vi "8通道控制_lock_in.vi"() -> ()   [LabVIEW 2021]
uses:
  <vilib>/Utility/error.llb/DialogType.ctl
  <vilib>/DAQmx/write.llb/DAQmx Write (Digital 2D U8 NChan NSamp).vi
  <vilib>/DAQmx/write.llb/DAQmx Write (Digital 2D U32 NChan NSamp).vi
  <vilib>/DAQmx/create/channels.llb/DAQmx Create Channel (DO-Digital Output).vi
  <vilib>/DAQmx/configure/timing.llb/DAQmx Timing (Sample Clock).vi
  <vilib>/DAQmx/miscellaneous.llb/DAQmx Fill In Error Info.vi
  <vilib>/DAQmx/configure/trigger.llb/DAQmx Start Trigger (Digital Edge).vi
  <vilib>/Utility/file.llb/Write Delimited Spreadsheet (DBL).vi
panel:
  out "error out":errorcluster
  out "写入时间（s)":dbl
  in  "采样率":dbl=10000000.0
  in  "保存总控件":bool
  in  "读取总控件":bool
  in  "Tab Control 2":enum32{"数字信号控制", "模拟信号控制"}(tab)
  out "运行状态-LED":bool
  out "运行状态":string
  in  "开始运行":bool
  in  "停止循环":bool
  in  "总时间 (ms)":dbl=100.0
  out "单通道总采样点":dbl=100000.0
  in  "结束运行":bool
  out "已运行时间 (s)":dbl
  in  "读取数字控件":bool
  in  "保存数字控件":bool
  in  "Port 0_0":T1
  out "运行状态1":bool
  in  "读取模拟控件":bool
  in  "保存模拟控件":bool
  in  "start":bool
  in  "stop":bool
  in  "Input":T2={"Digital Start Trigger Source 4"="/Dev1/PFI0", "Digital Start Trigger Edge 4"=10280, "min volt (V)"=-5.0, "max volt (V)"=5.0, "rate"=100000.0, "device name"="Dev1", "Formula In"=[], "Total time (s)"=0.0} {"rate" format="%0.2f"; "max volt (V)" format="%0.2f"; "min volt (V)" format="%0.2f"; "Digital Start Trigger Edge 4" items=["Rising"=10280, "Falling"=10171]}
  out "Output":T3={"Actual Rate"=0.0, "Actual SampPerChan"=0.0, "Mixed Signal Graph"=[], "模拟隔离器连接状态"="未连接模拟隔离器"}
  # "BEC时序控制程序"
  # "中山大学 量子工程与精密测量实验室 CPT信号控制系统"
  # "操作说明：\n1. 设置总时间和合适的采样率；\n2. 输入正数代表高电平的持续时间，负数对应低电平的持续时间。如少于总时间，之后默认为低电平；\n3. 可根据需要，拖动输入栏增加输入的时序数量；\n4. 模拟信号采用硬件触发，需将其中一个TTL信号（默认为P0.0）接入板卡的PFI0。\n5. 保存数据"
  # "AO Trigger"
  # "CPT/Probe"
  # "780"
  # "795"
  # "MOT-B"
  # "CCD"
  # "Bias-B"
  # "AI Trigger"
  # "1、Formula In 中 sample 为各个函数的持续时间\n2、Total time 为总时间，必须大于 sample 之和\n3、min volt 和 max volt 默认±10V\n4、rate 为采样率，即时钟频率\n5、device name 为选择的板卡，可选为 Dev1\n6、Source 为接受触发的端口，Edge 为触发类型"
  # "In0：780 VCO 幅值（初始 0.6）\nIn1：780 VCO 频率（初始 0.7）"
  # "Actual Rate 显示实际的时钟\n频率。Actual SampPer Chan显示\n每次采样的总样本点数。"
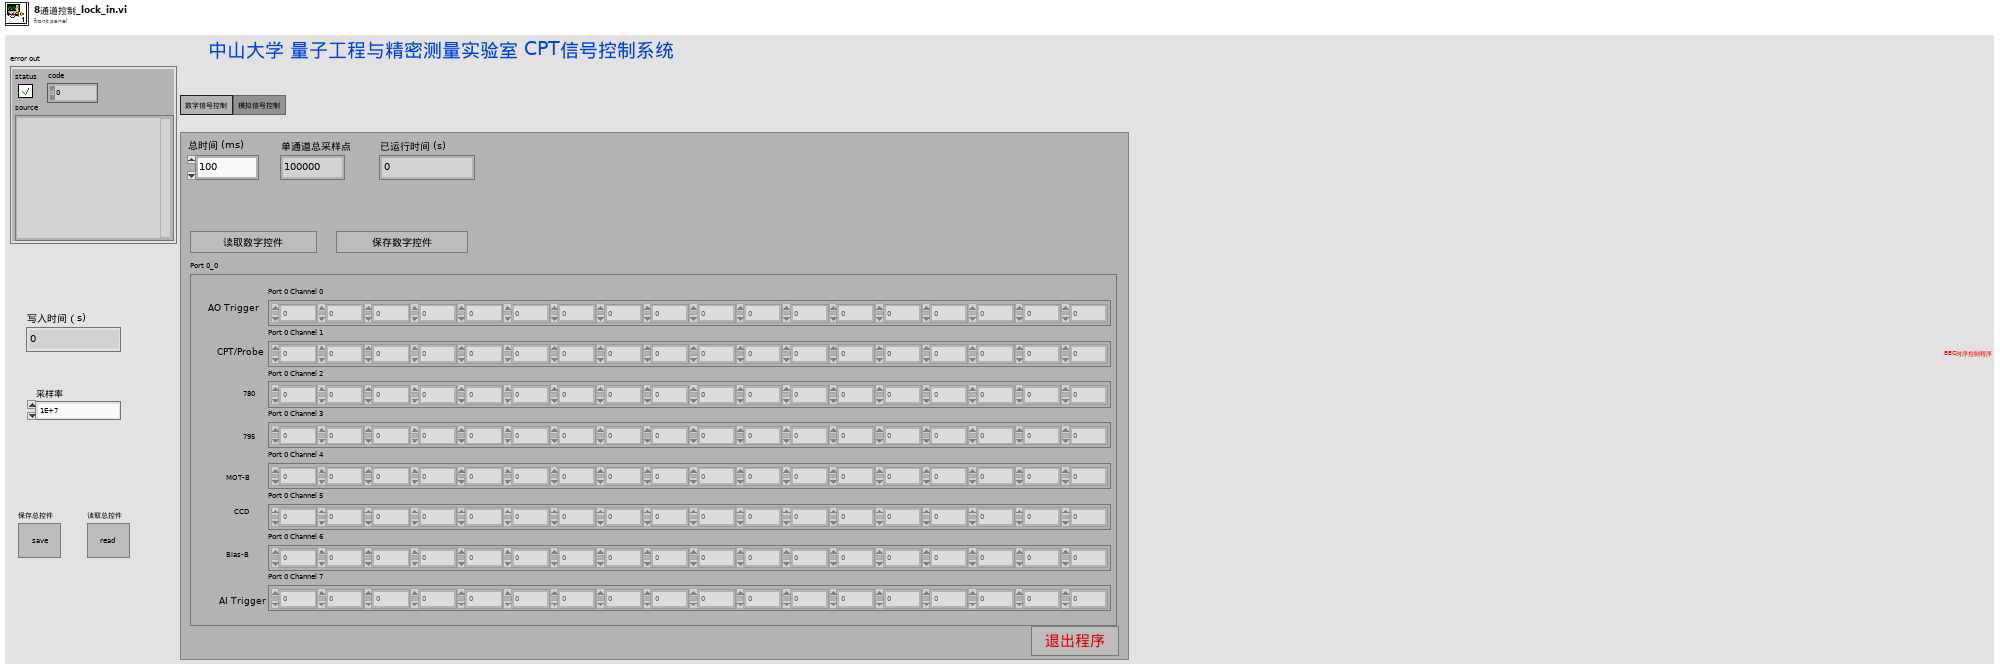
[diagram p1: front panel]
types:
  T1 = cluster{"Port 0 Channel 1":dbl[], "Port 0 Channel 2":dbl[], "Port 0 Channel 3":dbl[], "Port 0 Channel 4":dbl[], "Port 0 Channel 5":dbl[], "Port 0 Channel 6":dbl[], "Port 0 Channel 7":dbl[], "Port 0 Channel 0":dbl[]}
  T2 = cluster{"Digital Start Trigger Source 4":tag, "Digital Start Trigger Edge 4":i32, "min volt (V)":dbl, "max volt (V)":dbl, "rate":dbl, "device name":tag, "Formula In":cluster{" Sample1(s)":dbl, "formula1":string, "Sample2":dbl, "formula2":string, "Sample3":dbl, "formula3":string, "Sample4":dbl, "formula4":string}[], "Total time (s)":dbl}
  T3 = cluster{"Actual Rate":dbl, "Actual SampPerChan":dbl, "Mixed Signal Graph":waveform(dbl)[], "模拟隔离器连接状态":string}
  T4 = enum8{"Enabled", "Disabled", "Disabled and Grayed Out"}
  T5 = typedef "DialogType.ctl" = u16
  T6 = cluster{dbl[], dbl[], dbl[], dbl[], dbl[], dbl[], dbl[], dbl[]}
  T7 = cluster{"Digital Start Trigger Source 4":tag, "Digital Start Trigger Edge 4":i32, "minimum value":dbl, "maximum value":dbl, "rate":dbl, "device name":tag, "formular in":cluster{"Sample1":dbl, "formula1":string, "Sample2":dbl, "formula2":string, "Sample3":dbl, "formula3":string, "Sample4":dbl, "formula4":string}[], "Total time":dbl}
  T8 = cluster{"总时间 (ms)":dbl, "Port 0_0":cluster{"Port 0 Channel 1":dbl[], "Port 0 Channel 2":dbl[], "Port 0 Channel 3":dbl[], "Port 0 Channel 4":dbl[], "Port 0 Channel 5":dbl[], "Port 0 Channel 6":dbl[], "Port 0 Channel 7":dbl[], "Port 0 Channel 0":dbl[]}, "output":cluster{"Digital Start Trigger Source 4":string, "Digital Start Trigger Edge 4":string, "minimum value":dbl, "maximum value":dbl, "rate":dbl, "device name":string, "Total time":dbl, "Formula In":cluster{" Sample1(s)":dbl, "formula1":string, "Sample2":dbl, "formula2":string, "Sample3":dbl, "formula3":string, "Sample4":dbl, "formula4":string}[]}}
  T9 = cluster{"Digital Start Trigger Source 4":string, "Digital Start Trigger Edge 4":string, "minimum value":dbl, "maximum value":dbl, "rate":dbl, "device name":string, "Total time":dbl, "Formula In":cluster{" Sample1(s)":dbl, "formula1":string, "Sample2":dbl, "formula2":string, "Sample3":dbl, "formula3":string, "Sample4":dbl, "formula4":string}[]}
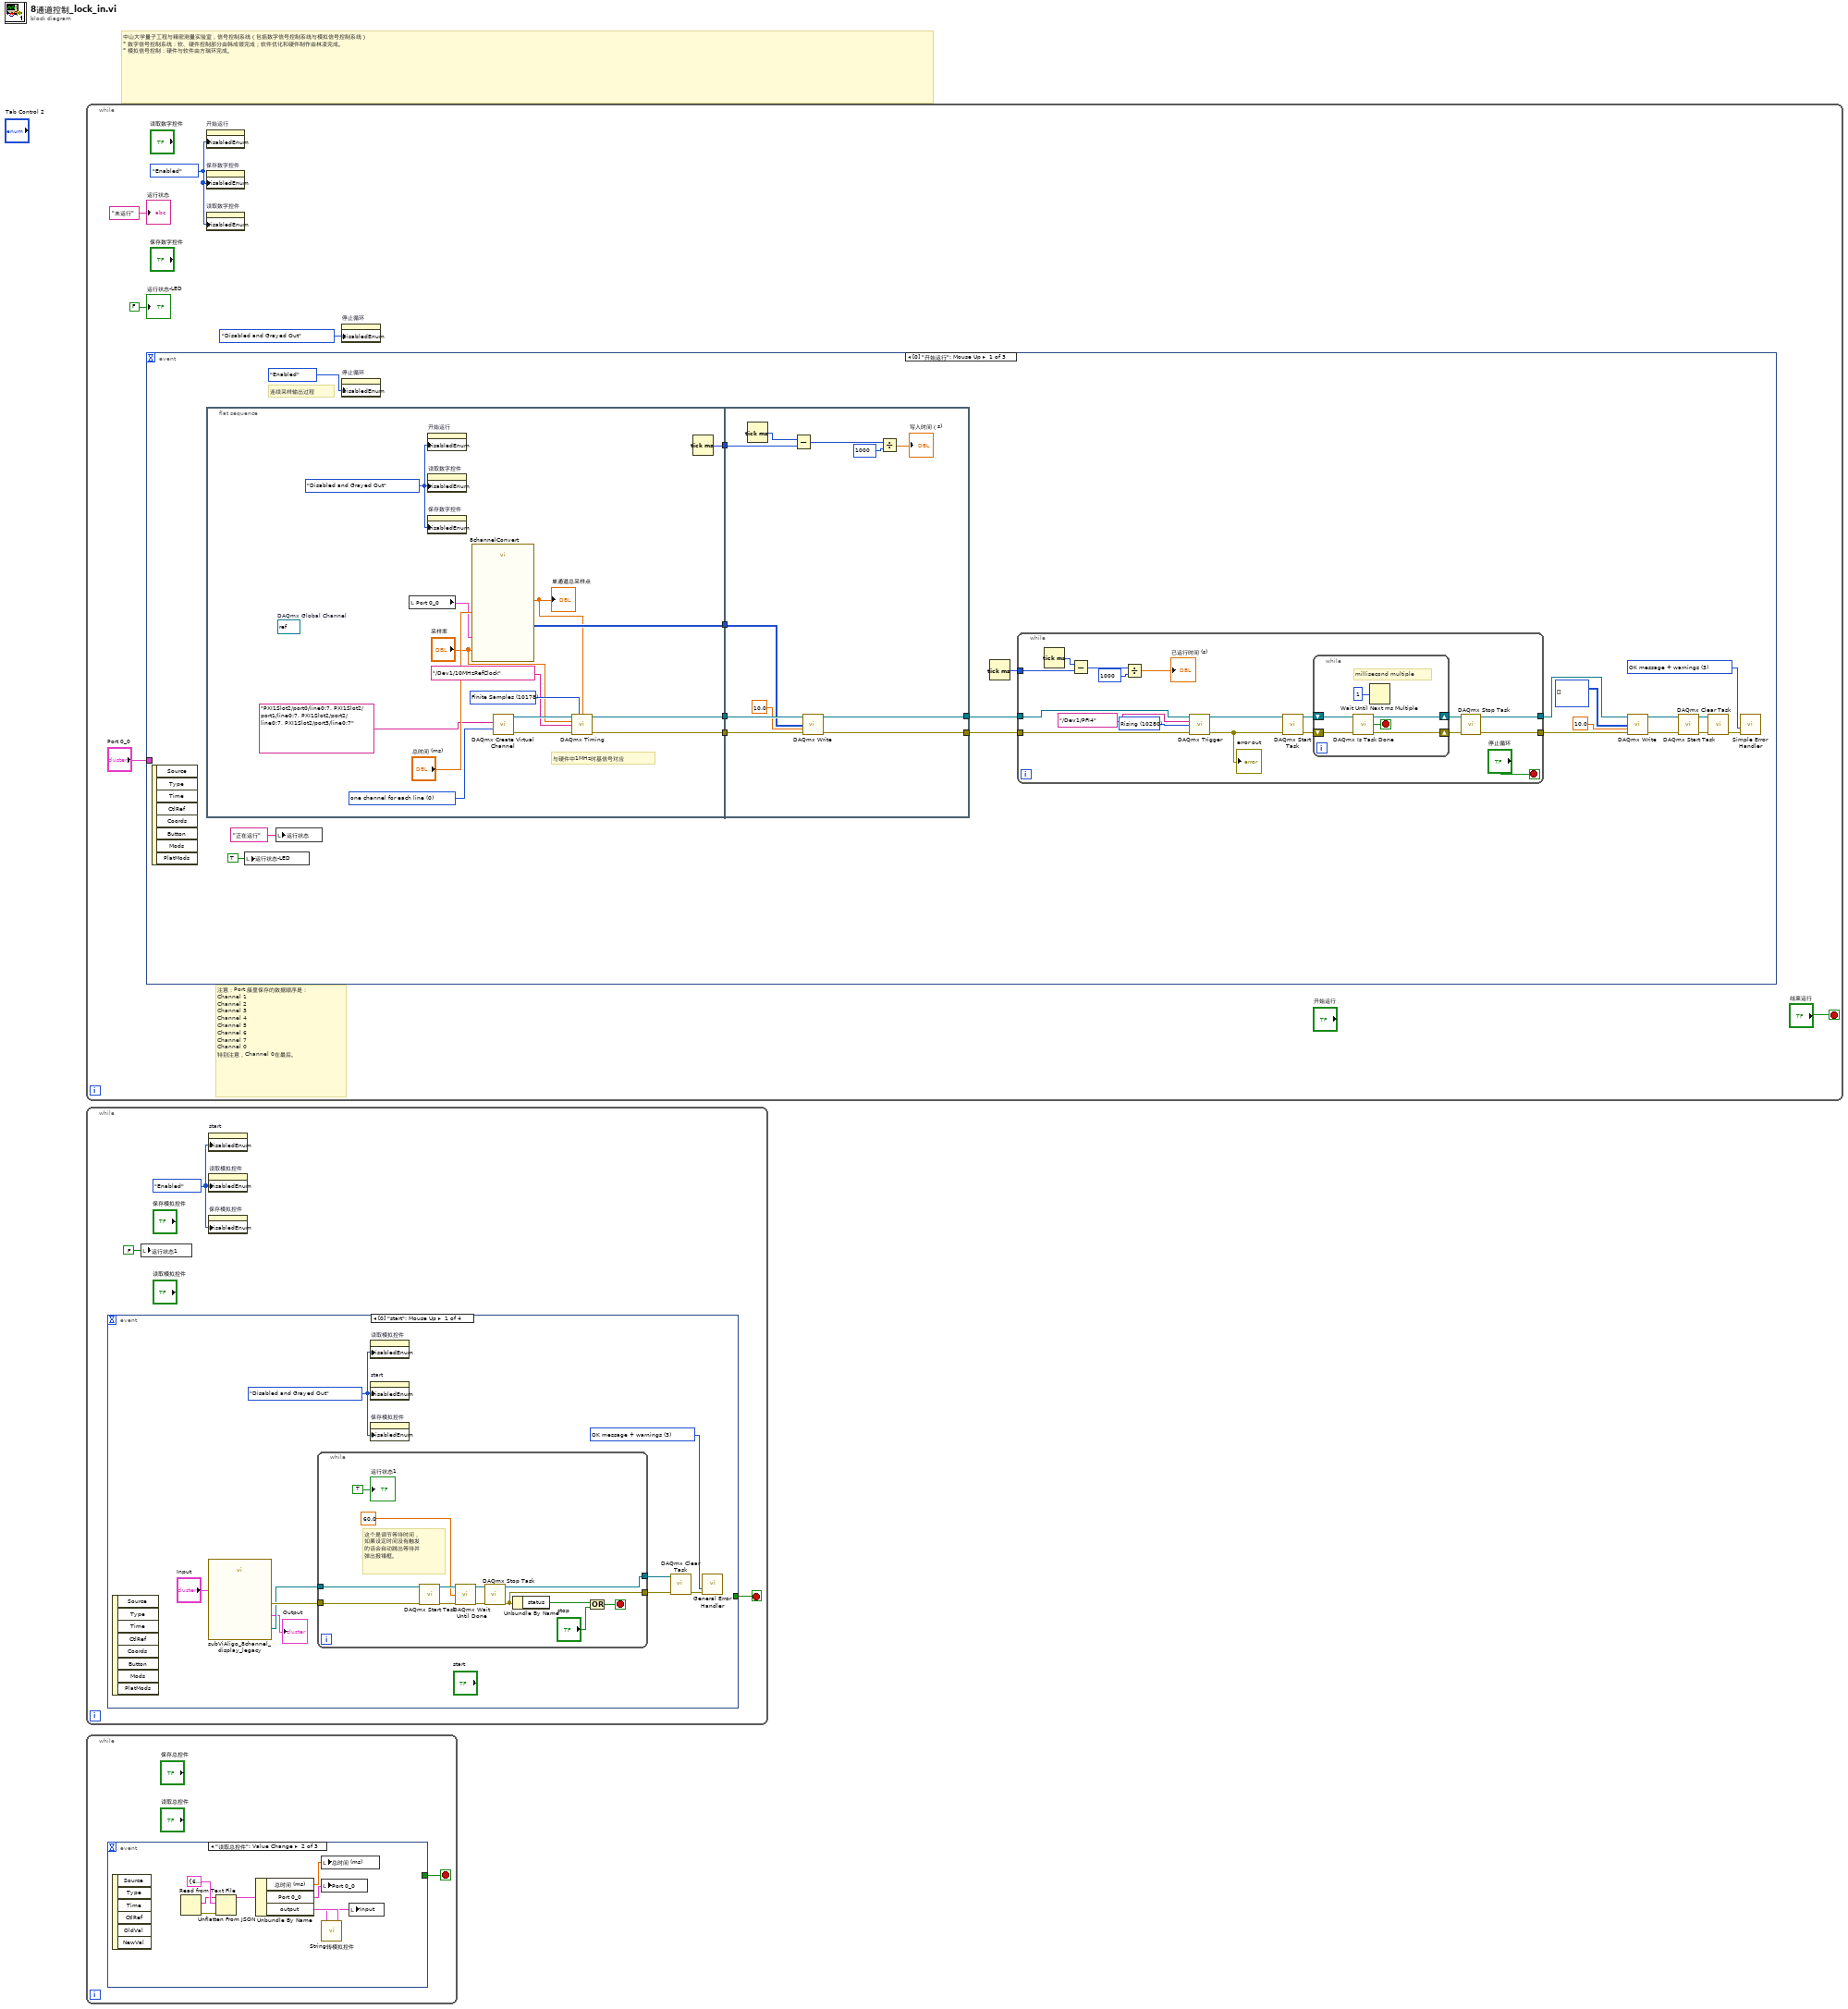
[diagram p0: block diagram]
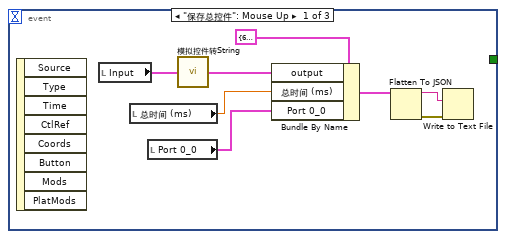
[diagram p2: hidden frame]
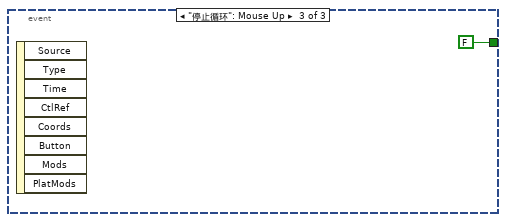
[diagram p3: hidden frame]
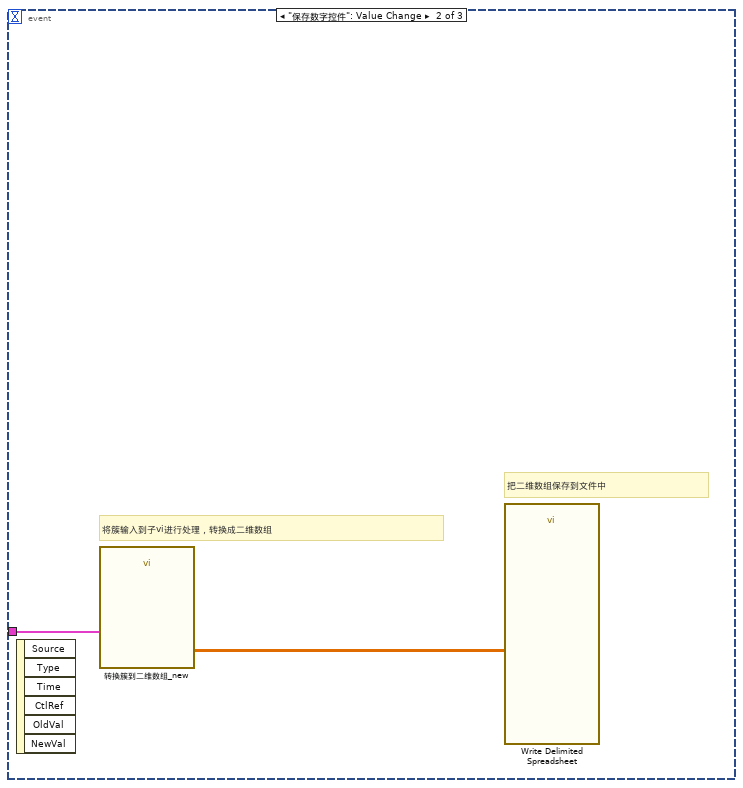
[diagram p4: hidden frame]
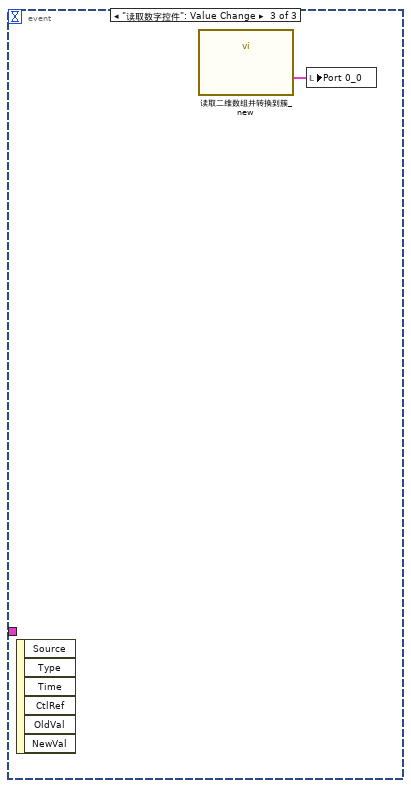
[diagram p5: hidden frame]
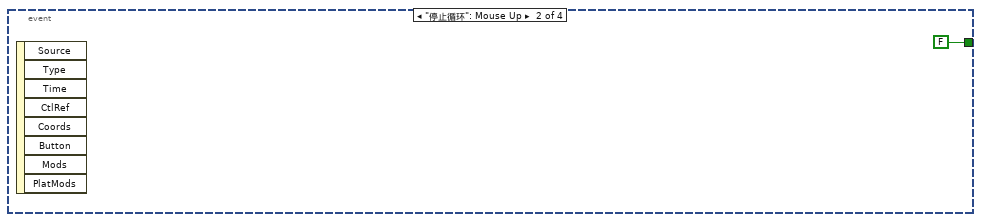
[diagram p6: hidden frame]
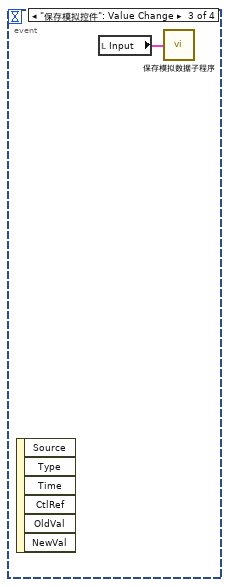
[diagram p7: hidden frame]
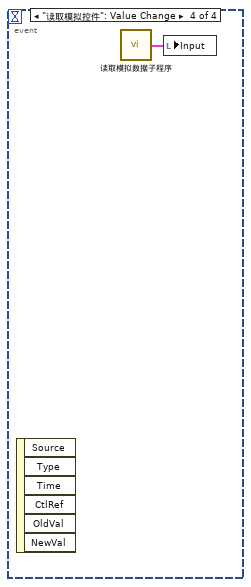
[diagram p8: hidden frame]
diagram:
  # "中山大学量子工程与精密测量实验室，信号控制系统（包括数字信号控制系统与模拟信号控制系统）\n* 数字信号控制系统：软、硬件控制部分由韩成银完成；软件优化和硬件制作由林凌完成。\n* 模拟信号控制：硬件与软件由方瑞环完成。"
  n1 = while {
    stop <- "结束运行" stop-if-true
    w1 = T4."Enabled" ("Disabled")
    # "注意：Port 簇里保存的数据顺序是：\nChannel 1\nChannel 2\nChannel 3\nChannel 4\nChannel 5\nChannel 6\nChannel 7\nChannel 0\n特别注意，Channel 0在最后。"
    n2 = event shown="[0] \"开始运行\": Mouse Up" {
      selector: _ -> [_ _ _]
      dyn-events: _ -> [_ _ _]
      timeout: _ -> [_ _ _]
      tunnel: "Port 0_0" -> [_ w77 _]
      event "开始运行": Mouse Up {
        w20 = T5 3 items=["no dialog", "OK message", "continue or stop message", "OK message + warnings", "continue/stop + warnings"] ("type of dialog (OK msg:1)")
        # "连续采样输出过程"
        n3 = event-data() -> ()  [unwired: 1 in, 8 out]
        n4 = flat-sequence {
          tunnel: [w37] -> w15
          tunnel: [w36] -> w14
          tunnel: [w34] -> w13
          tunnel: [w28] -> w12
          tunnel: w15 -> [w49]
          tunnel: w14 -> [w52]
          tunnel: w13 -> [w51]
          tunnel: [w43] -> w7
          tunnel: [w42] -> w8
          tunnel: w12 -> [w44]
          frame #0 {
            (unwired) refnum<k21> refnum  # DAQmx Global Channel
            w31 = T4."Disabled and Grayed Out" ("Disabled")
            w38 = 10178 items=["Finite Samples"=10178, "Continuous Samples"=10123, "Hardware Timed Single Point"=12522] ("sample mode")
            w41 = 0 items=["one channel for each line", "one channel for all lines"] ("line grouping")
            # "与硬件中1MHz时基信号对应"
            n5 = local read "Port 0_0"() -> (w30:T1)
            n6 = property on="开始运行" class="Bool"("DisabledEnum"=w31) -> ()  [unwired: 2 in, 2 out]
            n7 = property on="读取数字控件" class="Bool"("DisabledEnum"=w31) -> ()  [unwired: 2 in, 2 out]
            n8 = property on="保存数字控件" class="Bool"("DisabledEnum"=w31) -> ()  [unwired: 2 in, 2 out]
            n9 = call "8channelConvert.vi"("Port 0"=w30, "采样率"="采样率", "总时间（单位ms）"="总时间 (ms)") -> ("单通道总采样点"=w33:dbl, "appended array"=w34:u8[][])  [unwired: 23 in]
            "单通道总采样点" <- w33
            n10 = call-poly <vilib>:"DAQmx Create Virtual Channel.vi"("lines"=tag "PXI1Slot2/port0/line0:7, PXI1Slot2/port1/line0:7, PXI1Slot2/port2/line0:7, PXI1Slot2/port3/line0:7" ("Physical channels"), "line grouping"=w41) -> ("task out"=w40:refnum<k21>, "error out"=w39:errorcluster)  [unwired: 12 in]
            n11 = call-poly <vilib>:"DAQmx Timing.vi"("task/channels in"=w40, "sample mode"=w38, "samples per channel"=w33, "rate"="采样率", "source"=tag "/Dev1/10MHzRefClock", "error in"=w39) -> ("task out"=w36:refnum<k21>, "error out"=w37:errorcluster)  [unwired: 8 in]
            n12 = Tick Count (ms)() -> (millisecond timer value=w28:u32)
          }
          frame #1 {
            n13 = Tick Count (ms)() -> (millisecond timer value=w48:u32)
            n14 = Subtract(x=w48, y=w44) -> (x-y=w47:u32)
            n15 = call-poly <vilib>:"DAQmx Write.vi"("task/channels in"=w52, "data"=w51, "timeout"=10.0, "error in"=w49) -> ("task out"=w43:refnum<k21>, "error out"=w42:errorcluster)  [unwired: 9 in, 1 out]
            n16 = Divide(x=w47, y=u32 1000) -> (x/y=→"写入时间（s)":dbl)
          }
        }
        n17 = local write "运行状态-LED"(TRUE ("运行状态-LED 2")) -> ()
        n18 = local write "运行状态"("正在运行" ("运行状态 2")) -> ()
        n19 = property on="停止循环" class="Bool"("DisabledEnum"=T4."Enabled" ("Disabled")) -> ()  [unwired: 2 in, 2 out]
        n20 = Tick Count (ms)() -> (millisecond timer value=w17:u32)
        n21 = while {
          tunnel: w17 -> [w69]
          tunnel: [w62] -> w10
          tunnel: [w61] -> w9
          tunnel: w8 -> [w56]
          tunnel: w7 -> [w58]
          stop <- "停止循环" stop-if-true
          w54 = 10280 items=["Rising"=10280, "Falling"=10171] ("edge")
          n22 = Tick Count (ms)() -> (millisecond timer value=w70:u32)
          n23 = Subtract(x=w70, y=w69) -> (x-y=w68:u32)
          n24 = Divide(x=w68, y=u32 1000) -> (x/y=→"已运行时间 (s)":dbl)
          n25 = call-poly <vilib>:"DAQmx Trigger.vi"("task/channels in"=w58, "source"=tag "/Dev1/PFI4", "edge"=w54, "error in"=w56) -> ("task out"=w57:refnum<k21>, "error out"=w55:errorcluster)  [unwired: 10 in]
          "error out" <- w55
          n26 = call <vilib>:"DAQmx Start Task.vi"("task/channels in"=w57, "error in"=w55) -> ("task out"=w60:refnum<k21>, "error out"=w59:errorcluster)  [unwired: 12 in]
          n27 = while {
            shift-right: [w75] -> w64
            shift-left: w60 -> [w72]
            shift-right: [w74] -> w63
            shift-left: w59 -> [w71]
            stop <- w73 stop-if-true
            # "millisecond multiple"
            n28 = call <vilib>:"DAQmx Is Task Done.vi"("task/channels in"=w72, "error in"=w71) -> ("task out"=w75:refnum<k21>, "task done?"=w73:bool, "error out"=w74:errorcluster)  [unwired: 11 in]
            n29 = Wait Until Next ms Multiple(millisecond multiple=u32 1) -> ()  [unwired: 1 out]
          }
          n30 = call <vilib>:"DAQmx Stop Task.vi"("task/channels in"=w64, "error in"=w63) -> ("task out"=w62:refnum<k21>, "error out"=w61:errorcluster)  [unwired: 12 in]
        }
        n31 = call-poly <vilib>:"DAQmx Write.vi"("task/channels in"=w10, "data"=u8[][] [] ("appended array"), "timeout"=10.0, "error in"=w9) -> ("task out"=w25:refnum<k21>, "error out"=w24:errorcluster)  [unwired: 9 in, 1 out]
        n32 = call <vilib>:"DAQmx Start Task.vi"("task/channels in"=w25, "error in"=w24) -> ("task out"=w23:refnum<k21>, "error out"=w22:errorcluster)  [unwired: 12 in]
        n33 = call <vilib>:"DAQmx Clear Task.vi"("task in"=w23, "error in"=w22) -> ("error out"=w26:errorcluster)  [unwired: 13 in]
        n34 = call <vilib>:"Simple Error Handler.vi"("type of dialog (OK msg:1)"=w20, "error in (no error)"=w26) -> ()  [unwired: 3 in, 5 out]
      }
      event "保存数字控件": Value Change {
        # "把二维数组保存到文件中"
        # "将簇输入到子vi进行处理，转换成二维数组"
        n35 = event-data() -> ()  [unwired: 1 in, 6 out]
        n36 = call "转换簇到二维数组_new.vi"("Port 0"=w77) -> ("output 2D array"=w78:dbl[][])  [unwired: 10 in]
        n37 = call-poly <vilib>:"Write Delimited Spreadsheet.vi"("2D data"=w78) -> ()  [unwired: 13 in, 2 out]
      }
      event "读取数字控件": Value Change {
        n38 = event-data() -> ()  [unwired: 1 in, 6 out]
        n39 = call "读取二维数组并转换到簇_new.vi"() -> ("Port 0"=w79:T6)  [unwired: 11 in]
        n40 = local write "Port 0_0"(w79) -> ()
      }
    }
    n41 = property on="开始运行" class="Bool"("DisabledEnum"=w1) -> ()  [unwired: 2 in, 2 out]
    n42 = property on="保存数字控件" class="Bool"("DisabledEnum"=w1) -> ()  [unwired: 2 in, 2 out]
    n43 = property on="读取数字控件" class="Bool"("DisabledEnum"=w1) -> ()  [unwired: 2 in, 2 out]
    n44 = property on="停止循环" class="Bool"("DisabledEnum"=T4."Disabled and Grayed Out" ("Disabled")) -> ()  [unwired: 2 in, 2 out]
    "运行状态" <- "未运行" ("运行状态")
    "运行状态-LED" <- FALSE
  }
  n45 = while {
    stop <- w82 stop-if-true
    w80 = T4."Enabled" ("Disabled")
    n46 = event shown="[0] \"start\": Mouse Up" {
      selector: _ -> [_ _ _ _]
      dyn-events: _ -> [_ _ _ _]
      timeout: _ -> [_ _ _ _]
      tunnel: [_ FALSE _ _] -> w82
      event "start": Mouse Up {
        w84 = T4."Disabled and Grayed Out" ("Disabled")
        w91 = T5 3 items=["no dialog", "OK message", "continue or stop message", "OK message + warnings", "continue/stop + warnings"] ("type of dialog (OK msg:1)")
        n47 = event-data() -> ()  [unwired: 1 in, 8 out]
        n48 = call "subViAligo_8channel_display_legacy.vi"("Input"="Input") -> ("error out"=w87:errorcluster, "Output"=→"Output":T3, "task out"=w86:refnum<k21>)  [unwired: 4 in]
        n49 = while {
          tunnel: w86 -> [w103]
          tunnel: w87 -> [w102]
          tunnel: [w98] -> w89
          tunnel: [w97] -> w88
          stop <- w93 stop-if-true
          # "这个是调节等待时间，\n如果设定时间没有触发\n的话会自动跳出等待并\n弹出报错框。"
          n50 = call <vilib>:"DAQmx Start Task.vi"("task/channels in"=w103, "error in"=w102) -> ("task out"=w101:refnum<k21>, "error out"=w100:errorcluster)  [unwired: 12 in]
          n51 = call <vilib>:"DAQmx Wait Until Done.vi"("task/channels in"=w101, "timeout (sec)"=60.0, "error in"=w100) -> ("task out"=w99:refnum<k21>, "error out"=w104:errorcluster)  [unwired: 11 in]
          n52 = call <vilib>:"DAQmx Stop Task.vi"("task/channels in"=w99, "error in"=w104) -> ("task out"=w98:refnum<k21>, "error out"=w97:errorcluster)  [unwired: 12 in]
          n53 = Unbundle By Name(w97) -> ("status"=w95:bool)
          n54 = Or(x=w95, y="stop") -> (x .or. y?=w93:bool)
          "运行状态1" <- TRUE ("Boolean")
        }
        n55 = property on="读取模拟控件" class="Bool"("DisabledEnum"=w84) -> ()  [unwired: 2 in, 2 out]
        n56 = property on="start" class="Bool"("DisabledEnum"=w84) -> ()  [unwired: 2 in, 2 out]
        n57 = property on="保存模拟控件" class="Bool"("DisabledEnum"=w84) -> ()  [unwired: 2 in, 2 out]
        n58 = call <vilib>:"DAQmx Clear Task.vi"("task in"=w89, "error in"=w88) -> ("error out"=w90:errorcluster)  [unwired: 13 in]
        n59 = call <vilib>:"General Error Handler.vi"("type of dialog (OK msg:1)"=w91, "error in (no error)"=w90) -> ()  [unwired: 9 in, 5 out]
      }
      event "停止循环": Mouse Up {
        n60 = event-data() -> ()  [unwired: 1 in, 8 out]
      }
      event "保存模拟控件": Value Change {
        n61 = event-data() -> ()  [unwired: 1 in, 6 out]
        n62 = local read "Input"() -> (w106:T2)
        n63 = call "保存模拟数据子程序.vi"("Input"=w106) -> ()
      }
      event "读取模拟控件": Value Change {
        n64 = event-data() -> ()  [unwired: 1 in, 6 out]
        n65 = call "读取模拟数据子程序.vi"() -> ("Input"=w107:T7)
        n66 = local write "Input"(w107) -> ()
      }
    }
    n67 = local write "运行状态1"(FALSE ("Boolean")) -> ()
    n68 = property on="start" class="Bool"("DisabledEnum"=w80) -> ()  [unwired: 2 in, 2 out]
    n69 = property on="读取模拟控件" class="Bool"("DisabledEnum"=w80) -> ()  [unwired: 2 in, 2 out]
    n70 = property on="保存模拟控件" class="Bool"("DisabledEnum"=w80) -> ()  [unwired: 2 in, 2 out]
  }
  n71 = while {
    stop <- w108 stop-if-true
    n72 = event shown="[1] \"读取总控件\": Value Change" {
      selector: _ -> [_ _ _]
      dyn-events: _ -> [_ _ _]
      timeout: _ -> [_ _ _]
      tunnel: [_ _ FALSE] -> w108
      event "保存总控件": Mouse Up {
        n73 = event-data() -> ()  [unwired: 1 in, 8 out]
        n74 = local read "Input"() -> (w114:T2)
        n75 = local read "总时间 (ms)"() -> (w116:dbl)
        n76 = local read "Port 0_0"() -> (w115:T1)
        n77 = call "模拟控件转String.vi"("Input"=w114) -> ("output"=w112:T9)
        n78 = Bundle By Name(cluster=T8 {"总时间 (ms)"=6000.0, "Port 0_0"={"Port 0 Channel 1"=[], "Port 0 Channel 2"=[6000.0], "Port 0 Channel 3"=[6000.0], "Port 0 Channel 4"=[6000.0], "Port 0 Channel 5"=[], "Port 0 Channel 6"=[], "Port 0 Channel 7"=[], "Port 0 Channel 0"=[]}, "output"={"Digital Start Trigger Source 4"="/Dev1/PFI0", "Digital Start Trigger Edge 4"="", "minimum value"=-10.0, "maximum value"=10.0, "rate"=1000.0, "device name"="PXI1Slot5", "Total time"=0.0, "Formula In"=[]}}, "output"=w112, "总时间 (ms)"=w116, "Port 0_0"=w115) -> (w111:T8)
        n79 = Flatten To JSON(anything=w111) -> (JSON string=w109:string, 11:w110:errorcluster)  [unwired: 2 in]
        n80 = Write to Text File(text=w109, error in=w110) -> ()  [unwired: 2 in, 3 out]
      }
      event "读取总控件": Value Change {
        n81 = event-data() -> ()  [unwired: 1 in, 6 out]
        n82 = Read from Text File() -> (text=w123:string, error out=w122:errorcluster)  [unwired: 4 in, 2 out]
        n83 = Unflatten From JSON(JSON string=w123, type and defaults=T8 {"总时间 (ms)"=6000.0, "Port 0_0"={"Port 0 Channel 1"=[], "Port 0 Channel 2"=[6000.0], "Port 0 Channel 3"=[6000.0], "Port 0 Channel 4"=[6000.0], "Port 0 Channel 5"=[], "Port 0 Channel 6"=[], "Port 0 Channel 7"=[], "Port 0 Channel 0"=[]}, "output"={"Digital Start Trigger Source 4"="/Dev1/PFI0", "Digital Start Trigger Edge 4"="", "minimum value"=-10.0, "maximum value"=10.0, "rate"=1000.0, "device name"="PXI1Slot5", "Total time"=0.0, "Formula In"=[]}}, error in (no error)=w122) -> (value=w121:T8)  [unwired: 4 in, 1 out]
        n84 = Unbundle By Name(w121) -> ("总时间 (ms)"=w119:dbl, "Port 0_0"=w120:T1, "output"=w118:T9)
        n85 = local write "总时间 (ms)"(w119) -> ()
        n86 = local write "Port 0_0"(w120) -> ()
        n87 = call "String转模拟控件.vi"("output"=w118) -> ("Input"=w117:T2)
        n88 = local write "Input"(w117) -> ()
      }
      event "停止循环": Mouse Up {
        n89 = event-data() -> ()  [unwired: 1 in, 8 out]
      }
    }
  }
